vi "retrieve_vectors.vi"(0 "vector_qdrant in":refnum<class "vector_qdrant.lvclass">, 5 "colection_name":string, 7 "ids":string[](array[string]), 11 "error in (no error)":errorcluster) -> (4 "vector_qdrant out":refnum<class "vector_qdrant.lvclass">, 6 "Vectors":T1[](array[typedef]), 15 "error out":errorcluster)   [LabVIEW 2020, in "vector_qdrant.lvclass"]
uses:
  vector_qdrant.lvclass
  abstract_vector_base/vector.ctl
  vector_qdrant.lvclass/vector_qdrant.ctl
  <vilib>/httpClient/POSTBuffer.vi
  <vilib>/httpClient/LabVIEWHTTPClient.lvlib
  abstract_vector_base/abstract_vector_base.lvclass
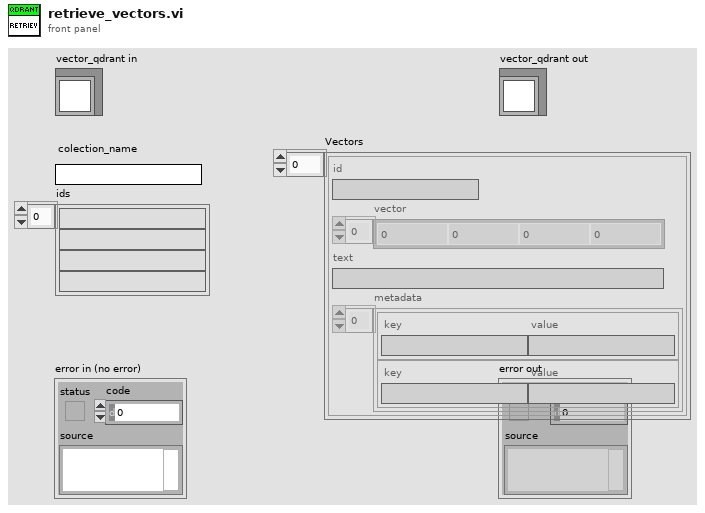
[diagram p1: front panel]
types:
  T1 = typedef "abstract_vector_base.lvclass/vector.ctl" = cluster{"id":string, "vector":dbl[], "text":string, "metadata":cluster{"key":string, "value":string}[]}
  T2 = cluster{"ids":string[], "with_payload":bool, "with_vector":bool}
  T3 = typedef "LabVIEWHTTPClient.lvlib/ClientHandle.ctl" = refnum<k1>
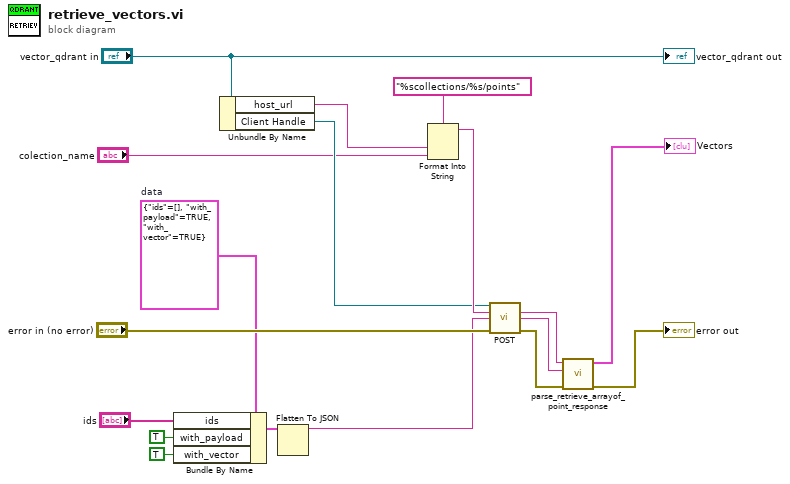
[diagram p0: block diagram]
diagram:
  w6 = T2 {"ids"=[], "with_payload"=TRUE, "with_vector"=TRUE}  # data
  n1 = Bundle By Name(cluster=w6, "ids"="ids", "with_payload"=TRUE, "with_vector"=TRUE) -> (w4:T2)
  n2 = Unbundle By Name("vector_qdrant in") -> ("host_url"=w13:string, "Client Handle"=w14:T3)
  n3 = Flatten To JSON(anything=w4) -> (JSON string=w3:string)  [unwired: 2 in, 1 out]
  n4 = Format Into String(format string="%scollections/%s/points", w13, "colection_name") -> (resulting string=w17:string)  [unwired: 2 in, 1 out]
  n5 = call-poly <vilib>:"POST.vi"("client handle"=w14, "url"=w17, "buffer"=w3, "error in (no error)"="error in (no error)") -> ("headers"=w11:string, "body"=w10:string, "error out"=w9:errorcluster)  [unwired: 8 in, 1 out]
  n6 = call "parse_retrieve_arrayof_point_response.vi"("error in (no error)"=w9, "body"=w10, "headers"=w11) -> ("error out"=→"error out":errorcluster, "Array"=→"Vectors":T1[])  [unwired: 7 in]
  "vector_qdrant out" <- "vector_qdrant in"
